vi "PLC设备连接.vi"(8 "error in (no error)":errorcluster caption="错误输入（无错误）", 11 "PLC设置":T1={"ActLogicalStationNumber"=9600, "ActUtlType"=refnum}) -> (0 "error out":errorcluster caption="错误输出", 2 "返回值":i32, 3 "PLC设置2":T1)   [LabVIEW 2015, in "Action.lvlib"]
uses:
  Action.lvlib
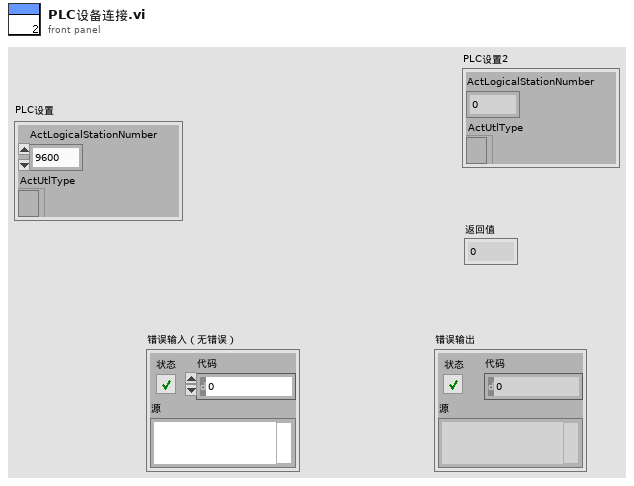
[diagram p1: front panel]
types:
  T1 = typedef "Action.lvlib/PLC设置.ctl" = cluster{"ActLogicalStationNumber":i32, "ActUtlType":refnum<k7>}
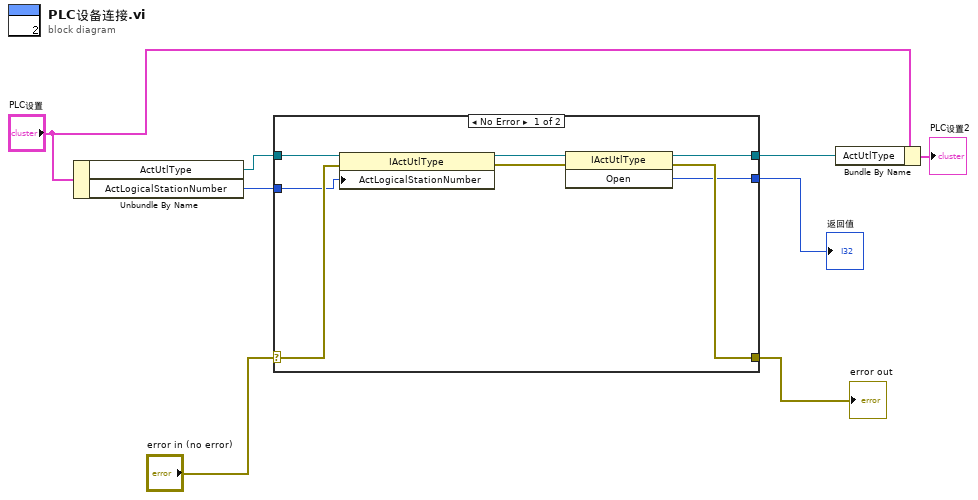
[diagram p0: block diagram]
diagram:
  n1 = Unbundle By Name("PLC设置") -> ("ActUtlType"=w4:refnum<k7>, "ActLogicalStationNumber"=w6:i32)
  n2 = case shown="No Error" "error in (no error)" {
    selector: "error in (no error)" -> [w15 w18]
    tunnel: [w11 w18] -> w7
    tunnel: w6 -> [w14 _]
    tunnel: w4 -> [w16 w17]
    tunnel: [w10 _] -> w5
    tunnel: [w9 w17] -> w2
    frame No Error {
      n3 = property class="IActUtlType"(reference=w16, error in=w15, "ActLogicalStationNumber"=w14) -> (reference out=w13:refnum<k7>, error out=w12:errorcluster)
      n4 = invoke class="IActUtlType" method="Open"(reference=w13, error in=w12) -> (reference out=w9:refnum<k7>, error out=w11:errorcluster, "Open"=w10:i32)  [unwired: 1 in]
    }
    frame Error {
    }
  }
  "error out" <- w7
  "返回值" <- w5
  n5 = Bundle By Name(cluster="PLC设置", "ActUtlType"=w2) -> (→"PLC设置2":T1)
